vi "read_error_message.vi"(8 "error in (no error)":errorcluster, 11 "ClientBuilder in":refnum<class "ClientBuilder.lvclass">) -> (0 "error out":errorcluster, 2 "error_message":string, 3 "ClientBuilder in":refnum<class "ClientBuilder.lvclass">)   [LabVIEW 2020, in "reqwest.lvlib" / "ClientBuilder.lvclass"]
uses:
  ClientBuilder.lvclass
  ClientBuilder.lvclass/ClientBuilder.ctl
  reqwest.lvlib
  lv_reqwest_64.dll
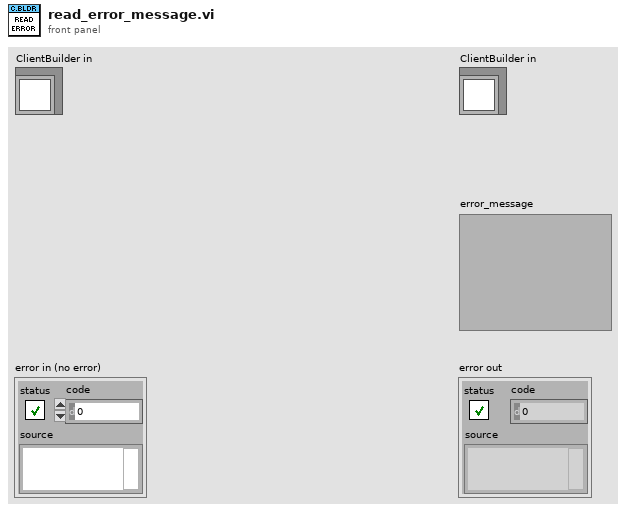
[diagram p1: front panel]
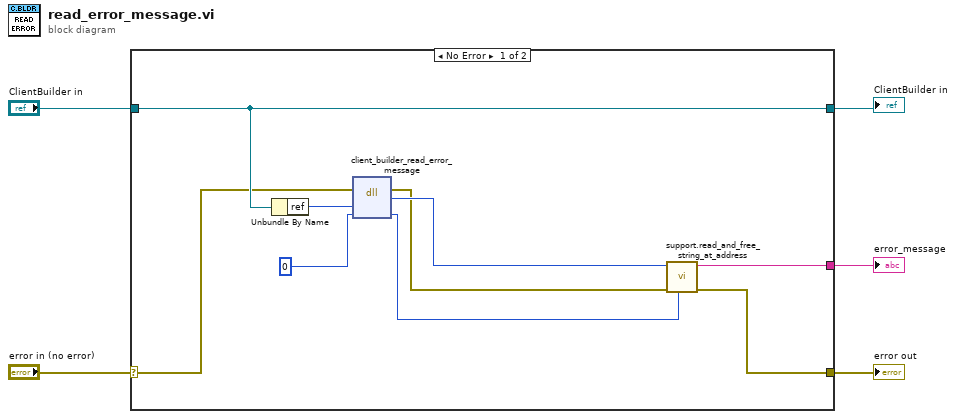
[diagram p0: block diagram]
diagram:
  n1 = case shown="No Error" "error in (no error)" {
    selector: "error in (no error)" -> [w9 w15]
    tunnel: "ClientBuilder in" -> [w10 w16]
    tunnel: [w11 _] -> w3
    tunnel: [w8 w15] -> w1
    tunnel: [w10 w16] -> w2
    frame No Error {
      n2 = Unbundle By Name(w10) -> ("ref"=w12:u64)
      n3 = dll-call lib="C:/Projects/vipm-desktop/source/submodules/reqwest-rs-labview/lv_src/lv_reqwest_*.*" fn="client_builder_read_error_message"(error in=w9, "request_id"=w12, "num_bytes"=u32 0) -> (error out=w13:errorcluster, "string_ptr"=w14:u64, "num_bytes"=w6:u32)  [unwired: 3 in, 1 out]
      n4 = call "support.read_and_free_string_at_address.vi"("string_length"=w6, "error in (no error)"=w13, "string_ptr"=w14) -> ("error out"=w8:errorcluster, "string"=w11:string)  [unwired: 7 in]
    }
    frame Error {
    }
  }
  "error out" <- w1
  "error_message" <- w3
  "ClientBuilder in" <- w2
